vi "onTestExecution.vi"(6 "timeout (2000 ms)":i32=2000, 7 "Name":string, 8 "error in (no error)":errorcluster, 11 "Test Runner.Library in":refnum<class "Test Runner.Library.lvclass">) -> (0 "error out":errorcluster, 3 "Test Runner.Library out":refnum<class "Test Runner.Library.lvclass">)   [LabVIEW 2013, in "Caraya.lvlib" / "Test Runner.Library.lvclass"]
uses:
  Test Runner.Library.lvclass
  Test Runner/Test Runner.lvclass
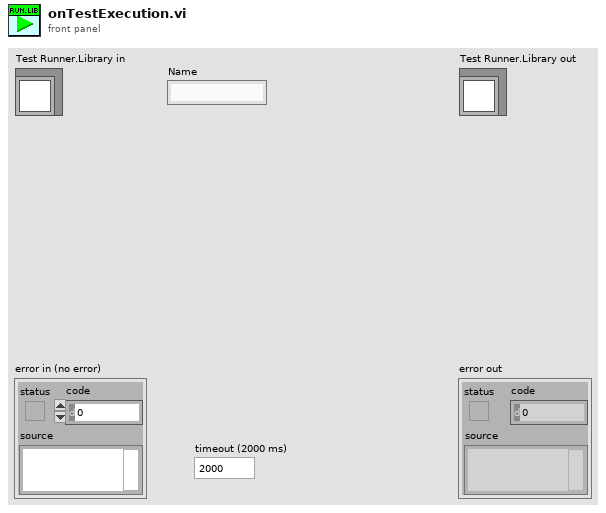
[diagram p1: front panel]
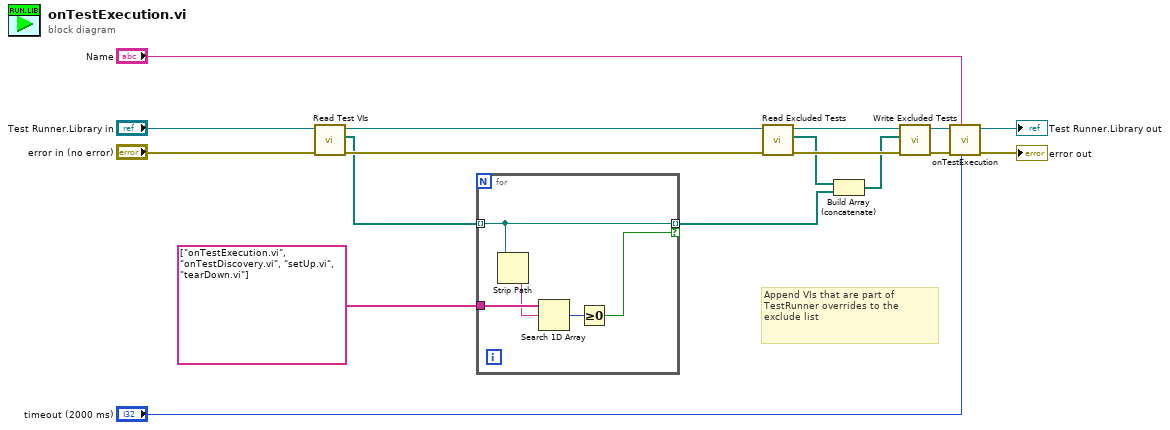
[diagram p0: block diagram]
diagram:
  # "Append VIs that are part of TestRunner overrides to the exclude list"
  n1 = call "Read Test VIs.vi"("error in (no error)"="error in (no error)", "Test Runner in"="Test Runner.Library in") -> ("error out"=w12:errorcluster, "Test VIs"=w9:path[], "Test Runner out"=w13:refnum<class "Test Runner.Library.lvclass">)  [unwired: 7 in]
  n2 = for {
    tunnel: w9 -> [w22] mode=indexing
    tunnel: [w22] -> w8 mode=indexing if=w18
    tunnel: string[] ["onTestExecution.vi", "onTestDiscovery.vi", "setUp.vi", "tearDown.vi"] -> [w21]
    n3 = Strip Path(path=w22) -> (name=w20:string)  [unwired: 1 out]
    n4 = Search 1D Array(1D array=w21, element=w20) -> (index of element=w19:i32)  [unwired: 1 in]
    n5 = Greater Or Equal To 0?(x=w19) -> (x >= 0?=w18:bool)
  }
  n6 = call "Read Excluded Tests.vi"("error in (no error)"=w12, "Test Runner in"=w13) -> ("error out"=w17:errorcluster, "Excluded Tests"=w11:path[], "Test Runner out"=w15:refnum<class "Test Runner.Library.lvclass">)  [unwired: 7 in]
  n7 = Build Array (concatenate)(w11, w8) -> (w10:path[])
  n8 = call "Write Excluded Tests.vi"("error in (no error)"=w17, "Excluded Tests"=w10, "Test Runner in"=w15) -> ("error out"=w16:errorcluster, "Test Runner out"=w14:refnum<class "Test Runner.Library.lvclass">)  [unwired: 7 in]
  n9 = call-parent "onTestExecution.vi"("timeout (2000 ms)"="timeout (2000 ms)", "Name"="Name", "error in (no error)"=w16, "Test Runner in"=w14) -> ("error out"=→"error out":errorcluster, "Test Runner out"=→"Test Runner.Library out":refnum<class "Test Runner.Library.lvclass">)  [unwired: 6 in]
